vi "Rayon transcript.vi"() -> ()   [LabVIEW 2017]
panel:
  out "x .and. y?":u16
  out "D Float out":sgl
  out "Int_F":bool
  out "D Int out":i32
  out "idx o":u8
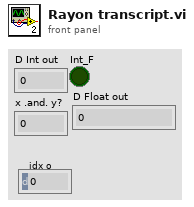
[diagram p1: front panel]
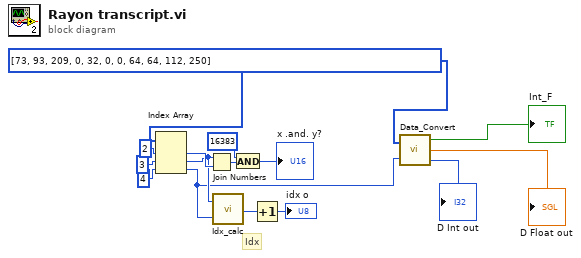
[diagram p0: block diagram]
diagram:
  w6 = u8[] [73, 93, 209, 0, 32, 0, 0, 64, 64, 112, 250]
  # "Idx"
  n1 = Index Array(array=w6, index #1=2 ("index"), index #2=3 ("index"), index #3=4 ("index")) -> (element #1=w13:u8, element #2=w9:u8, element #3=w5:u8)
  n2 = Join Numbers(hi=w9, lo=w13) -> ((hi.lo)=w11:u16)
  n3 = call "Idx_calc.vi"("bit4"=w5, "bit3"=w9) -> ("idx"=w7:u8)
  n4 = And(x=u16 16383, y=w11) -> (x .and. y?=→"x .and. y?":u16)
  n5 = Increment(x=w7) -> (x+1=→"idx o":u8)
  n6 = call "Data_Convert.vi"("Data Type"=w5, "Array"=w6) -> ("D Int out"=→"D Int out":i32, "D Float out"=→"D Float out":sgl, "Int_F"=→"Int_F":bool)
